vi "SR_FlipFlop.vi"(2 "R":bool, 3 "CLK":bool, 4 "S":bool) -> (0 "__\nQ":bool, 1 "Q":bool)   [LabVIEW 2018]
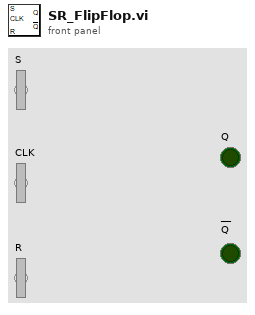
[diagram p1: front panel]
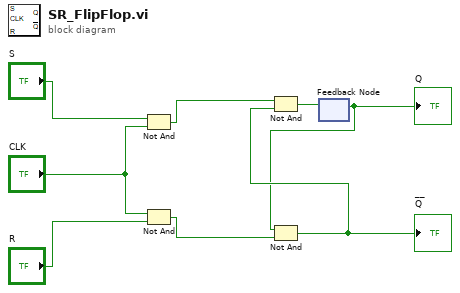
[diagram p0: block diagram]
diagram:
  n1 = Not And(1:"CLK", 2:"S") -> (0:w5:bool)
  n2 = Not And(1:"R", 2:"CLK") -> (0:w4:bool)
  n3 = feedback #1() -> (w1:bool)  [unwired: 1 in]
  "Q" <- w1
  n4 = Not And(1:w4, 2:w1) -> (0:w3:bool)
  "__\nQ" <- w3
  n5 = Not And(1:w3, 2:w5) -> (0:w2:bool)
  n6 = feedback-in #1(w2) -> ()
